vi "Pump Action-Status.vi"(8 "error in (no error)":errorcluster, 10 "Message Data":variant, 11 "Data Cluster":T1 {"Pump Info"."Direction" items=["CW", "CCW"]; "Pump Info"."Speed" format="%03.0f"}) -> (0 "error out":errorcluster, 3 "Data Cluster out":T1 {"Pump Info"."Direction" items=["CW", "CCW"]; "Pump Info"."Speed" format="%03.0f"})   [LabVIEW 2020, in "Pump.lvlib"]
uses:
  Pump.lvlib
  Pump Hardware Configuration.ctl
  support/Message Queue/Message Cluster.ctl
  support/Message Queue/Message Queue.lvlib
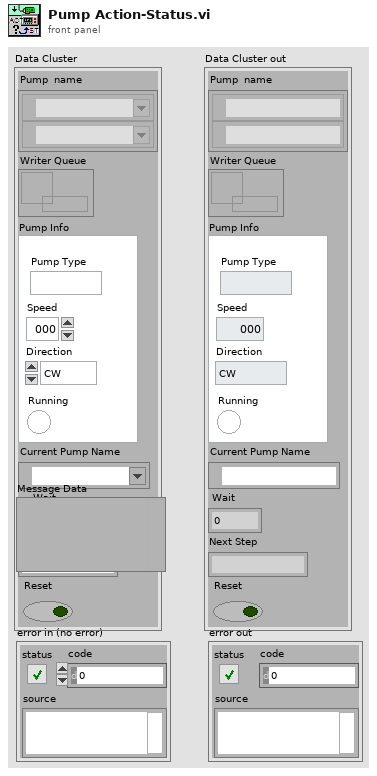
[diagram p1: front panel]
types:
  T1 = typedef "Pump.lvlib/Pump Hardware Configuration.ctl" = cluster{"Pump  name":refnum<visa-resource-name>[], "Writer Queue":refnum<queue>, "Pump Info":cluster{"Pump Type":string, "Speed":i32, "Direction":u16, "Running":bool}, "Current Pump Name":refnum<visa-resource-name>, "Wait":dbl, "Next Step":string, "Reset":bool}
  T2 = typedef "Message Queue.lvlib/Message Cluster.ctl" = cluster{"Message":string, "Message Data":variant}
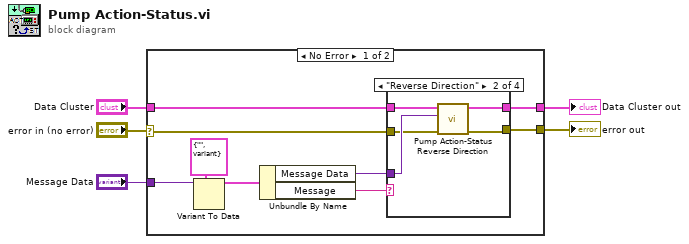
[diagram p0: block diagram]
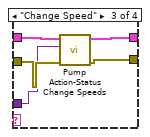
[diagram p3: hidden frame]
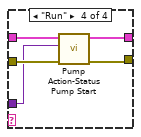
[diagram p4: hidden frame]
diagram:
  n1 = case shown="No Error" "error in (no error)" {
    selector: "error in (no error)" -> [w7 w32]
    tunnel: [w14 w32] -> w5
    tunnel: "Data Cluster" -> [w13 w33]
    tunnel: [w12 w33] -> w3
    tunnel: "Message Data" -> [w8 _]
    frame No Error {
      n2 = Variant To Data(type=T2 {"Message"="", "Message Data"=variant} ("element"), Variant=w8) -> (data=w10:T2)  [unwired: 1 in, 1 out]
      n3 = Unbundle By Name(w10) -> ("Message Data"=w6:variant, "Message"=w11:string)
      n4 = case shown="\"Reverse Direction\"" w11 {
        tunnel: w6 -> [_ w18 w22 w28]
        tunnel: [w16 w19 w25 w30] -> w12
        tunnel: w13 -> [w16 w20 w26 w31]
        tunnel: w7 -> [w15 w17 w23 w29]
        tunnel: [w15 w21 w24 w27] -> w14
        frame "False", Default {
        }
        frame "Reverse Direction" {
          n5 = call "Pump Action-Status Reverse Direction.vi"("error in (no error)"=w17, "Message Data"=w18, "Data Cluster in"=w20) -> ("error out"=w21:errorcluster, "Data Cluster out"=w19:T1)  [unwired: 7 in]
        }
        frame "Change Speed" {
          n6 = call "Pump Action-Status Change Speeds.vi"("error in (no error)"=w23, "Message Data"=w22, "Data Cluster in"=w26) -> ("error out"=w24:errorcluster, "Data Cluster out"=w25:T1)  [unwired: 7 in]
        }
        frame "Run" {
          n7 = call "Pump Action-Status Pump Start.vi"("error in (no error)"=w29, "Message Data"=w28, "Data Cluster in"=w31) -> ("error out"=w27:errorcluster, "Data Cluster out"=w30:T1)  [unwired: 7 in]
        }
      }
    }
    frame Error {
    }
  }
  "error out" <- w5
  "Data Cluster out" <- w3
